vi "Rohde & Schwarz VNA Set External Trigger Mode.vi"(6 "Channel":i8=1 min=1 max=99 step=1, 7 "Rohde & Schwarz VNA":T1, 8 "error in (no error)":errorcluster, 10 "Ext. Trigger Mode":T2, 11 "VISA Resource Name":refnum<visa-resource-name>) -> (0 "error out":errorcluster, 3 "dup VISA Resource Name":refnum<visa-resource-name>)   [LabVIEW 2011]
doc: "This VI for the HP8753B Network Analyzers reads the stimulus values. Except when performing log sweeps and freq list sweeps, this VI uses the start and stop values and the number of points to calcuate the stimulus values."
uses:
  TypeDefs/Rohde & Schwarz VNA External Trigger Mode.ctl
  TypeDefs/Rohde & Schwarz VNA Instrument Info.ctl
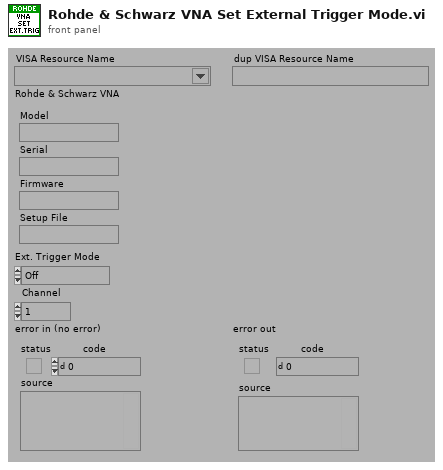
[diagram p1: front panel]
types:
  T1 = typedef "Rohde & Schwarz VNA Instrument Info.ctl" = cluster{"Model":string, "Serial":string, "Firmware":string, "Setup File":string}
  T2 = typedef "Rohde & Schwarz VNA External Trigger Mode.ctl" = enum16{"Off", "Rising Edge", "Falling Edge", "Periodic", "Manual"}
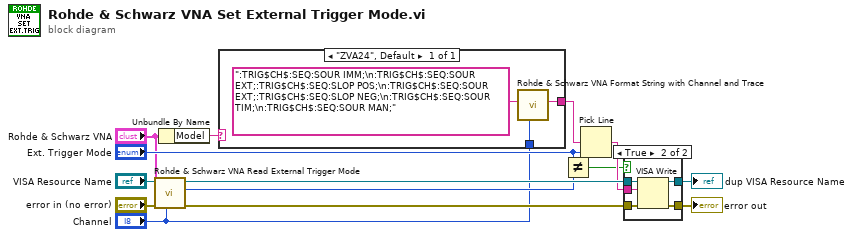
[diagram p0: block diagram]
diagram:
  n1 = call "Rohde & Schwarz VNA Read External Trigger Mode.vi"("Channel"="Channel", "Rohde & Schwarz VNA"="Rohde & Schwarz VNA", "error in (no error)"="error in (no error)", "VISA Resource Name"="VISA Resource Name") -> ("error out"=w9:errorcluster, "Ext. Trigger Mode"=w7:T2, "dup VISA Resource Name"=w8:refnum<visa-resource-name>)  [unwired: 5 out]
  n2 = Unbundle By Name("Rohde & Schwarz VNA") -> ("Model"=w2:string)
  n3 = case shown="\"ZVA24\", Default" w2 {
    tunnel: [w16] -> w5
    tunnel: "Channel" -> [w15]
    frame "ZVA24", Default {
      n4 = call "Rohde & Schwarz VNA Format String with Channel and Trace.vi"("Channel"=w15, "String"=":TRIG$CH$:SEQ:SOUR IMM;\n:TRIG$CH$:SEQ:SOUR EXT;:TRIG$CH$:SEQ:SLOP POS;\n:TRIG$CH$:SEQ:SOUR EXT;:TRIG$CH$:SEQ:SLOP NEG;\n:TRIG$CH$:SEQ:SOUR TIM;\n:TRIG$CH$:SEQ:SOUR MAN;") -> ("String Out"=w16:string)  [unwired: 1 in, 6 out]
    }
  }
  n5 = Not Equal?(x="Ext. Trigger Mode", y=w7) -> (x != y?=w4:bool)
  n6 = Pick Line(multi-line string=w5, line index="Ext. Trigger Mode") -> (output string=w6:string)  [unwired: 1 out]
  n7 = case shown="True" w4 {
    tunnel: w9 -> [w18 w24]
    tunnel: w8 -> [w19 w23]
    tunnel: w6 -> [_ w22]
    tunnel: [w19 w21] -> w14
    tunnel: [w18 w20] -> w13
    frame False {
    }
    frame True {
      n8 = VISA Write(VISA resource name=w23, write buffer=w22, error in (no error)=w24) -> (VISA resource name out=w21:refnum<visa-resource-name>, error out=w20:errorcluster)  [unwired: 1 out]
    }
  }
  "dup VISA Resource Name" <- w14
  "error out" <- w13
